vi "setValue.vi"(8 "error in (no error)":errorcluster, 10 "Value":bool, 11 "tBSONBoolean in":refnum<class "tBSONBoolean.lvclass">) -> (0 "error out":errorcluster, 3 "tBSONBoolean out":refnum<class "tBSONBoolean.lvclass">)   [LabVIEW 2013, in "BSON.lvlib" / "tBSONBoolean.lvclass"]
uses:
  tBSONBoolean.lvclass
  tBSONBoolean.lvclass/tBSONBoolean.ctl
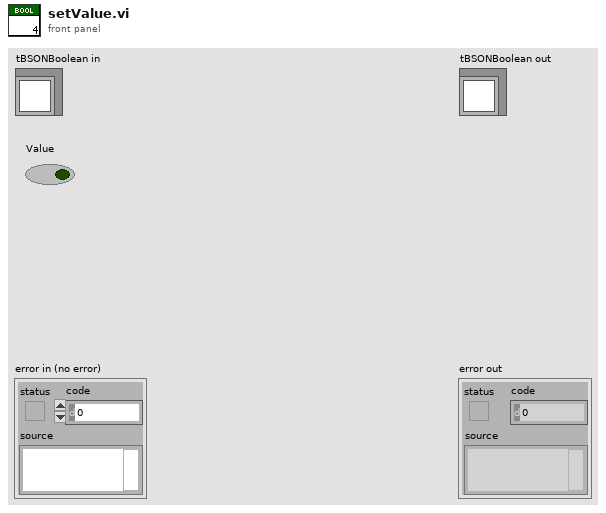
[diagram p1: front panel]
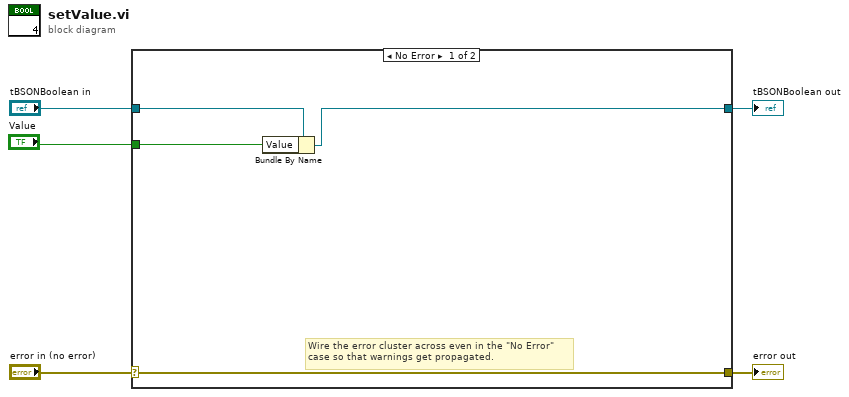
[diagram p0: block diagram]
diagram:
  n1 = case shown="No Error" "error in (no error)" {
    selector: "error in (no error)" -> [w9 w11]
    tunnel: [w9 w11] -> w4
    tunnel: [w6 w10] -> w2
    tunnel: "tBSONBoolean in" -> [w8 w10]
    tunnel: "Value" -> [w7 _]
    frame No Error {
      # "Wire the error cluster across even in the \"No Error\"\ncase so that warnings get propagated."
      n2 = Bundle By Name(cluster=w8, "Value"=w7) -> (w6:refnum<class "tBSONBoolean.lvclass">)
    }
    frame Error {
    }
  }
  "error out" <- w4
  "tBSONBoolean out" <- w2
